vi "VdLaser_Implement.vi"(11 "ClassThatImplements":refnum<class "VdLaser.lvclass">) -> (3 "InterfaceHelpClass":refnum<class "VdLaser_MyINterface.lvclass">)   [LabVIEW 2010, in "VdLaser_MyINterface.lvclass"]
doc: "Implemnts an Interface"
uses:
  VdLaser_MyINterface.lvclass
  VdLaser_class/VdLaser.lvclass
  VdLaser_MyINterface.lvclass/VdLaser_MyINterface.ctl
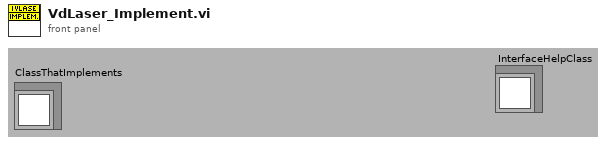
[diagram p1: front panel]
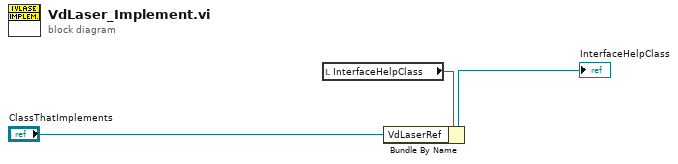
[diagram p0: block diagram]
diagram:
  n1 = local read "InterfaceHelpClass"() -> (w1:refnum<class "VdLaser_MyINterface.lvclass">)
  n2 = Bundle By Name(cluster=w1, "VdLaserRef"="ClassThatImplements") -> (→"InterfaceHelpClass":refnum<class "VdLaser_MyINterface.lvclass">)
